vi "Event Structure String Count word 6.vi"() -> ()   [LabVIEW 2020]
panel:
  out "Total Word":i32
  out "length":i32
  in  "String":string
  in  "Stop":bool
  # "Event Structure String : Count Word"
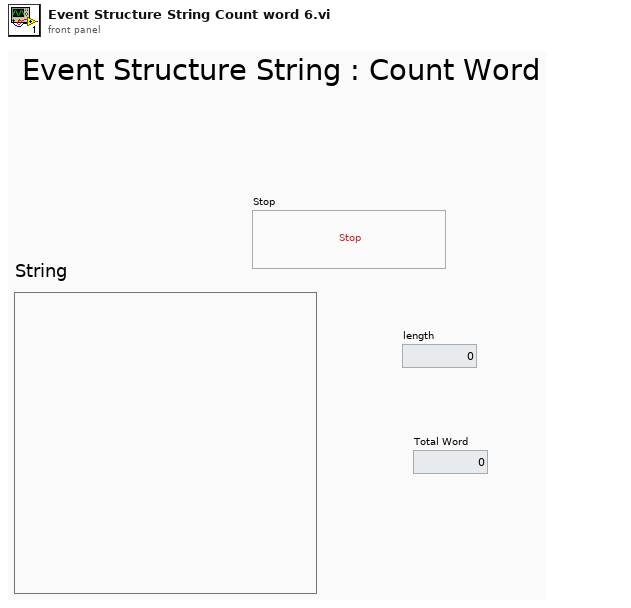
[diagram p1: front panel]
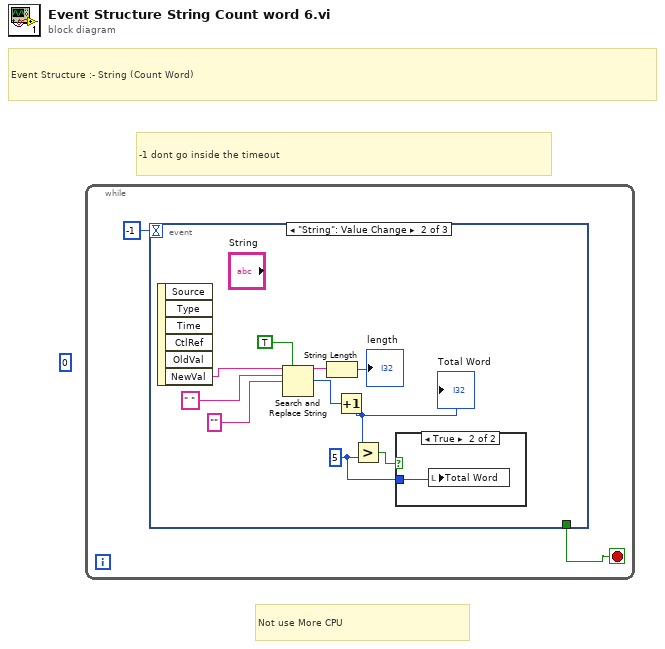
[diagram p0: block diagram]
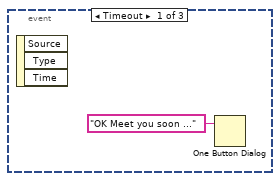
[diagram p2: hidden frame]
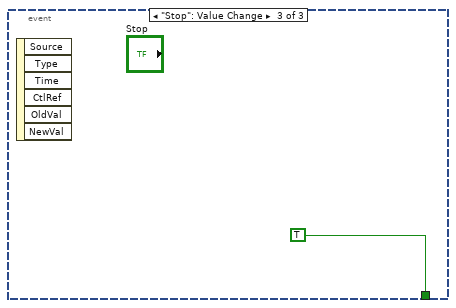
[diagram p4: hidden frame]
diagram:
  (unwired) 0
  # "Not use More CPU"
  # "-1 dont go inside the timeout"
  # "Event Structure :- String (Count Word)"
  n1 = while {
    stop <- w1 stop-if-true
    n2 = event shown="[1] \"String\": Value Change" {
      selector: _ -> [_ _ _]
      dyn-events: _ -> [_ _ _]
      timeout: -1 -> [_ _ _]
      tunnel: [_ _ TRUE] -> w1
      event Timeout {
        n3 = event-data() -> ()  [unwired: 1 in, 3 out]
        n4 = One Button Dialog(message="OK Meet you soon ...") -> ()  [unwired: 1 in, 1 out]
      }
      event "String": Value Change {
        w4 = 5 ("y")
        n5 = event-data() -> ("NewVal"=w13:string)  [unwired: 1 in, 5 out]
        n6 = Search and Replace String(replace all?=TRUE ("replace all? (F)"), input string=w13, search string=" ", replace string="" ("replace string (\"\")")) -> (result string=w10:string, number of replacements=w7:i32)  [unwired: 4 in, 2 out]
        n7 = String Length(string=w10) -> (length=→"length":i32)
        n8 = Increment(x=w7) -> (x+1=w6:i32)
        "Total Word" <- w6
        n9 = Greater?(x=w6, y=w4) -> (0:w5:bool)
        n10 = case shown="True" w5 {
          tunnel: w4 -> [_ w14]
          frame False {
          }
          frame True {
            n11 = local write "Total Word"(w14) -> ()
          }
        }
      }
      event "Stop": Value Change {
        n12 = event-data() -> ()  [unwired: 1 in, 6 out]
      }
    }
  }
